vi "CTIFF Writing Example.vi"() -> ()   [LabVIEW 8.6]
uses:
  ctiff.llb/__CTIFFNewFileAndStyleUINT16.vi
  ctiff.llb/__CTIFFAddNewPageUINT16.vi
panel:
  in  "Metadata":string[](array[string])
  in  "Name Tag":string
  in  "Image Description":string
  in  "Software":string
  in  "Camera Model":string
  in  "Camera Make":string
  in  "Copyright":string
  in  "Artist":string
  out "error":errorcluster
  in  "Pages":i32
  in  "Image":u16[][](array[numeric])
  in  "output file":path
  # "Required image data"
  # "Option data to add to each image"
  # "Extended Metadata"
  # "Basic Metadata"
  # "CamTIFF"
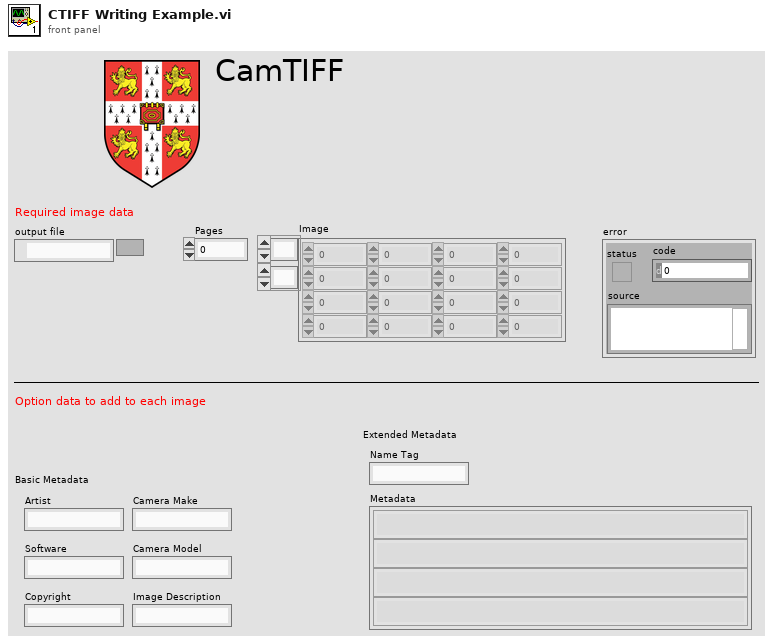
[diagram p1: front panel]
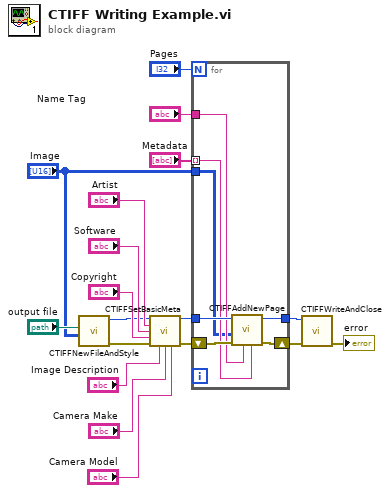
[diagram p0: block diagram]
diagram:
  n1 = call-poly "CTIFFNewFileAndStyle.vi"("image"="Image", "output_file"="output file") -> ("error"=w6:errorcluster, "CTIFF"=w5:i64)  [unwired: 8 in]
  n2 = call "CTIFFSetBasicMeta.vi"("CTIFF"=w5, "artist"="Artist", "software"="Software", "copyright"="Copyright", "error"=w6, "image description"="Image Description", "camera maker"="Camera Make", "camera model"="Camera Model") -> ("CTIFF"=w12:i64, "error"=w4:errorcluster)  [unwired: 6 in]
  n3 = for {
    N: "Pages" -> [_]
    tunnel: "Name Tag" -> [w22]
    tunnel: "Image" -> [w19]
    tunnel: "Metadata" -> [w21] mode=indexing
    tunnel: w12 -> [w25]
    shift-right: [w23] -> w3
    shift-left: w4 -> [w24]
    tunnel: [w20] -> w1
    n4 = call-poly "CTIFFAddNewPage.vi"("Extended Metadata"=w21, "Key for Extended Metadata"=w22, "error"=w24, "image"=w19, "CTIFF"=w25) -> ("error"=w23:errorcluster, "CTIFF"=w20:i64)  [unwired: 5 in]
  }
  n5 = call "CTIFFWriteAndClose.vi"("error"=w3, "CTIFF"=w1) -> ("error"=→"error":errorcluster)  [unwired: 9 in]
